vi "getRequestedStatus.vi"(8 "error in (no error)":errorcluster, 11 "AndorIKonAcquisitor in":refnum<class "AndorIKonAcquisitor.lvclass">) -> (0 "error out":errorcluster, 2 "String":string, 3 "AndorIKonAcquisitor out":refnum<class "AndorIKonAcquisitor.lvclass">)   [LabVIEW 2011, in "Hardware.lvlib" / "Channels.lvlib" / "AndorIKonAcquisitor.lvclass"]
uses:
  AndorIKonAcquisitor.lvclass
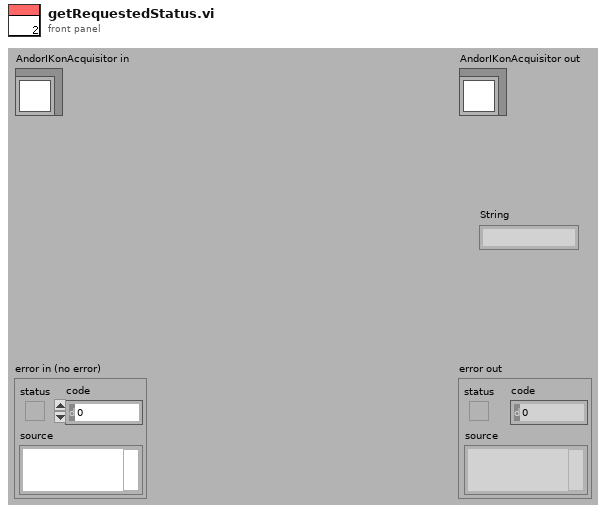
[diagram p1: front panel]
types:
  T1 = typedef "Error Code Enum typedef.ctl" = enum32{"N/A (0)", "DRV_ERROR_CODES", "DRV_SUCCESS", "DRV_VXDNOTINSTALLED", "DRV_ERROR_SCAN", "DRV_ERROR_CHECK_SUM", "DRV_ERROR_FILELOAD", "DRV_UNKNOWN_FUNC", "DRV_ERROR_VXD_INIT", "DRV_ERROR_ADDRESS", "DRV_ERROR_PAGELOCK", "DRV_ERROR_PAGEUNLOCK", "DRV_ERROR_BOARDTEST", "DRV_ERROR_ACK", "DRV_ERROR_UP_FIFO", "DRV_ERROR_PATTERN", "N/A (16)", "DRV_ACQUISITION_ERRORS", "DRV_ACQ_BUFFER", "DRV_ACQ_DOWNFIFO_FULL", "DRV_PROC_UNKONWN_INSTRUCTION", "DRV_ILLEGAL_OP_CODE", "DRV_KINETIC_TIME_NOT_MET", "DRV_ACCUM_TIME_NOT_MET", "DRV_NO_NEW_DATA", "N/A (25)", "DRV_SPOOLERROR", "N/A (27)", "N/A (28)", "N/A (29)", "N/A (30)", "N/A (31)", "N/A (32)", "DRV_TEMPERATURE_CODES", "DRV_TEMPERATURE_OFF", "DRV_TEMPERATURE_NOT_STABILIZED", "DRV_TEMPERATURE_STABILIZED", "DRV_TEMPERATURE_NOT_REACHED", "DRV_TEMPERATURE_OUT_RANGE", "DRV_TEMPERATURE_NOT_SUPPORTED", "DRV_TEMPERATURE_DRIFT", "N/A (41)", "N/A (42)", "N/A (43)", "N/A (44)", "N/A (45)", "N/A (46)", "N/A (47)", "N/A (48)", "DRV_GENERAL_ERRORS", "DRV_INVALID_AUX", "DRV_COF_NOTLOADED", "DRV_FPGAPROG", "DRV_FLEXERROR", "DRV_GPIBERROR", "N/A (55)", "N/A (56)", "N/A (57)", "N/A (58)", "N/A (59)", "N/A (60)", "N/A (61)", "N/A (62)", "N/A (63)", "DRV_DATATYPE", "DRV_DRIVER_ERRORS", "DRV_P1INVALID", "DRV_P2INVALID", "DRV_P3INVALID", "DRV_P4INVALID", "DRV_INIERROR", "DRV_COFERROR", "DRV_ACQUIRING", "DRV_IDLE", "DRV_TEMPCYCLE", "DRV_NOT_INITIALIZED", "DRV_P5INVALID", "DRV_P6INVALID", "DRV_INVALID_MODE", "DRV_INVALID_FILTER", "DRV_I2CERRORS", "DRV_I2CDEVNOTFOUND", "DRV_I2CTIMEOUT", "DRV_P7INVALID", "N/A (84)", "N/A (85)", "N/A (86)", "N/A (87)", "N/A (88)", "N/A (89)", "DRV_IOCERROR", "DRV_VRMVERSIONERROR"}
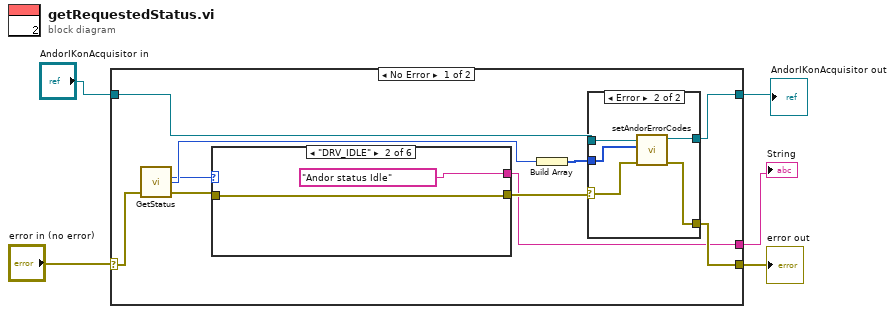
[diagram p0: block diagram]
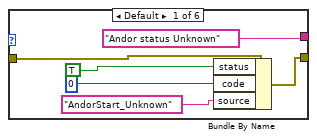
[diagram p2: hidden frame]
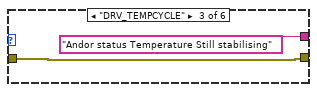
[diagram p3: hidden frame]
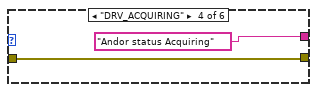
[diagram p4: hidden frame]
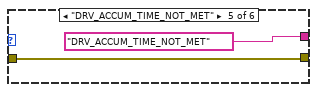
[diagram p5: hidden frame]
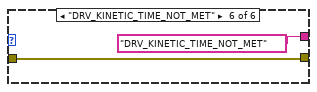
[diagram p6: hidden frame]
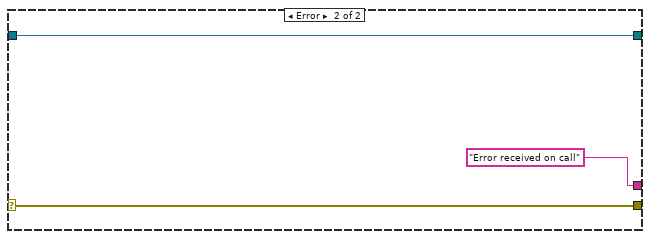
[diagram p8: hidden frame]
diagram:
  n1 = case shown="No Error" "error in (no error)" {
    selector: "error in (no error)" -> [w11 w41]
    tunnel: "AndorIKonAcquisitor in" -> [w14 w40]
    tunnel: [w13 w40] -> w5
    tunnel: [w12 w41] -> w2
    tunnel: [w6 "Error received on call"] -> w1
    frame No Error {
      n2 = call <userlib>:"GetStatus.vi"("error in (no error)"=w11) -> ("error out"=w9:errorcluster, "DLL error code"=w8:u32, "status"=w7:T1)  [unwired: 2 in]
      n3 = case shown="\"DRV_IDLE\"" w7 {
        tunnel: [w17 w23 w24 w27 w29 w31] -> w15
        tunnel: w9 -> [w18 w23 w24 w27 w29 w31]
        tunnel: ["Andor status Unknown" "Andor status Idle" "Andor status Temperature Still stabilising" "Andor status Acquiring" "DRV_ACCUM_TIME_NOT_MET" "DRV_KINETIC_TIME_NOT_MET"] -> w6
        frame Default {
          n4 = Bundle By Name(cluster=w18, "status"=TRUE, "code"=0, "source"="AndorStart_Unknown") -> (w17:errorcluster)
        }
        frame "DRV_IDLE" {
        }
        frame "DRV_TEMPCYCLE" {
        }
        frame "DRV_ACQUIRING" {
        }
        frame "DRV_ACCUM_TIME_NOT_MET" {
        }
        frame "DRV_KINETIC_TIME_NOT_MET" {
        }
      }
      n5 = Build Array(w8) -> (w10:u32[])
      n6 = case shown="Error" w15 {
        selector: w15 -> [w33 w37]
        tunnel: w14 -> [w32 w38]
        tunnel: [w32 w35] -> w13
        tunnel: [w33 w36] -> w12
        tunnel: w10 -> [_ w34]
        frame No Error {
        }
        frame Error {
          n7 = call-dynamic "setAndorErrorCodes.vi"("error in (no error)"=w37, "Andor Error Codes"=w34, "AndorIKonAcquisitor.lvclass in"=w38) -> ("error out"=w36:errorcluster, "AndorIKonAcquisitor.lvclass out"=w35:refnum<class "AndorIKonAcquisitor.lvclass">)  [unwired: 7 in]
        }
      }
    }
    frame Error {
    }
  }
  "error out" <- w2
  "AndorIKonAcquisitor out" <- w5
  "String" <- w1
